vi "Convert Data to Offset values.vi"(11 "Messages":T1(array[cluster])) -> (2 "all values":sgl[](array[numeric]), 3 "Values":string)   [LabVIEW 2025]
uses:
  Station/Controls/Offset_Values.ctl
panel:
  out "Offset F":sgl
  out "Offset E":sgl
  out "Offset D":sgl
  out "Diff Volt F":sgl
  out "Diff Volt E":sgl
  out "Diff Volt D":sgl
  out "Offset A":sgl
  out "Offset B":sgl
  out "Offset C":sgl
  out "Diff Volt C":sgl
  out "Diff Volt B":sgl
  out "Diff Volt A":sgl
  out "OffsetHiBrdgVolt":sgl
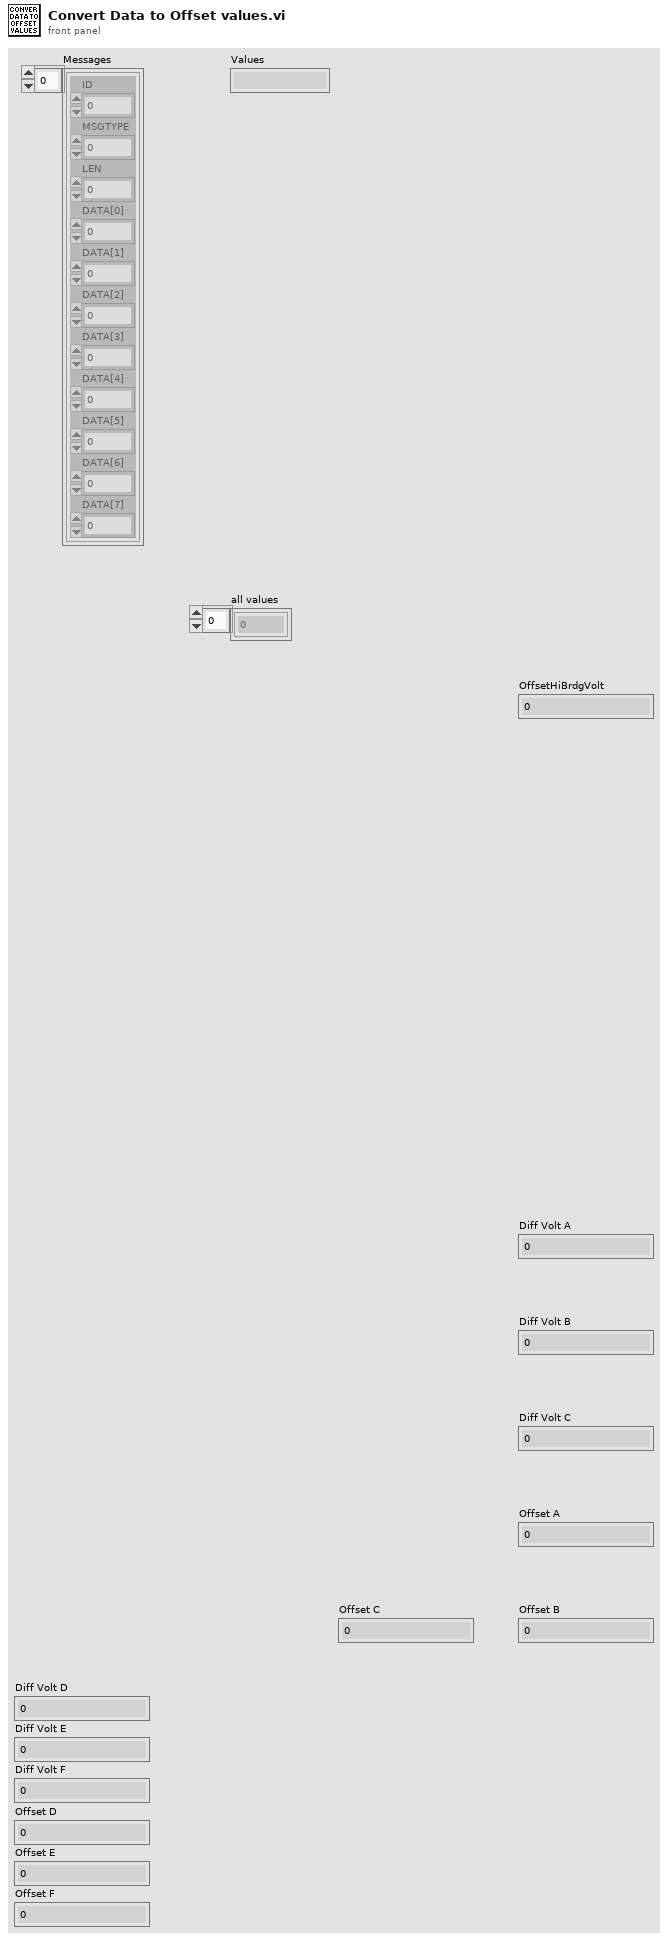
[diagram p1: front panel]
types:
  T1 = cluster{"ID":u32, "MSGTYPE":u8, "LEN":u8, "DATA[0]":u8, "DATA[1]":u8, "DATA[2]":u8, "DATA[3]":u8, "DATA[4]":u8, "DATA[5]":u8, "DATA[6]":u8, "DATA[7]":u8}[]
  T2 = cluster{"ID":u32, "MSGTYPE":u8, "LEN":u8, "DATA[0]":u8, "DATA[1]":u8, "DATA[2]":u8, "DATA[3]":u8, "DATA[4]":u8, "DATA[5]":u8, "DATA[6]":u8, "DATA[7]":u8}
  T3 = typedef "Offset_Values.ctl" = cluster{"OffsetHiBrdgVolt":sgl, "Diff Volt A ":sgl, "Diff Volt B":sgl, "Diff Volt C":sgl, "Diff Volt D":sgl, "Diff Volt E":sgl, "Diff Volt F":sgl, "Offset A":sgl, "Offset B":sgl, "Offset C":sgl, "Offset D":sgl, "Offset E":sgl, "Offset F":sgl}
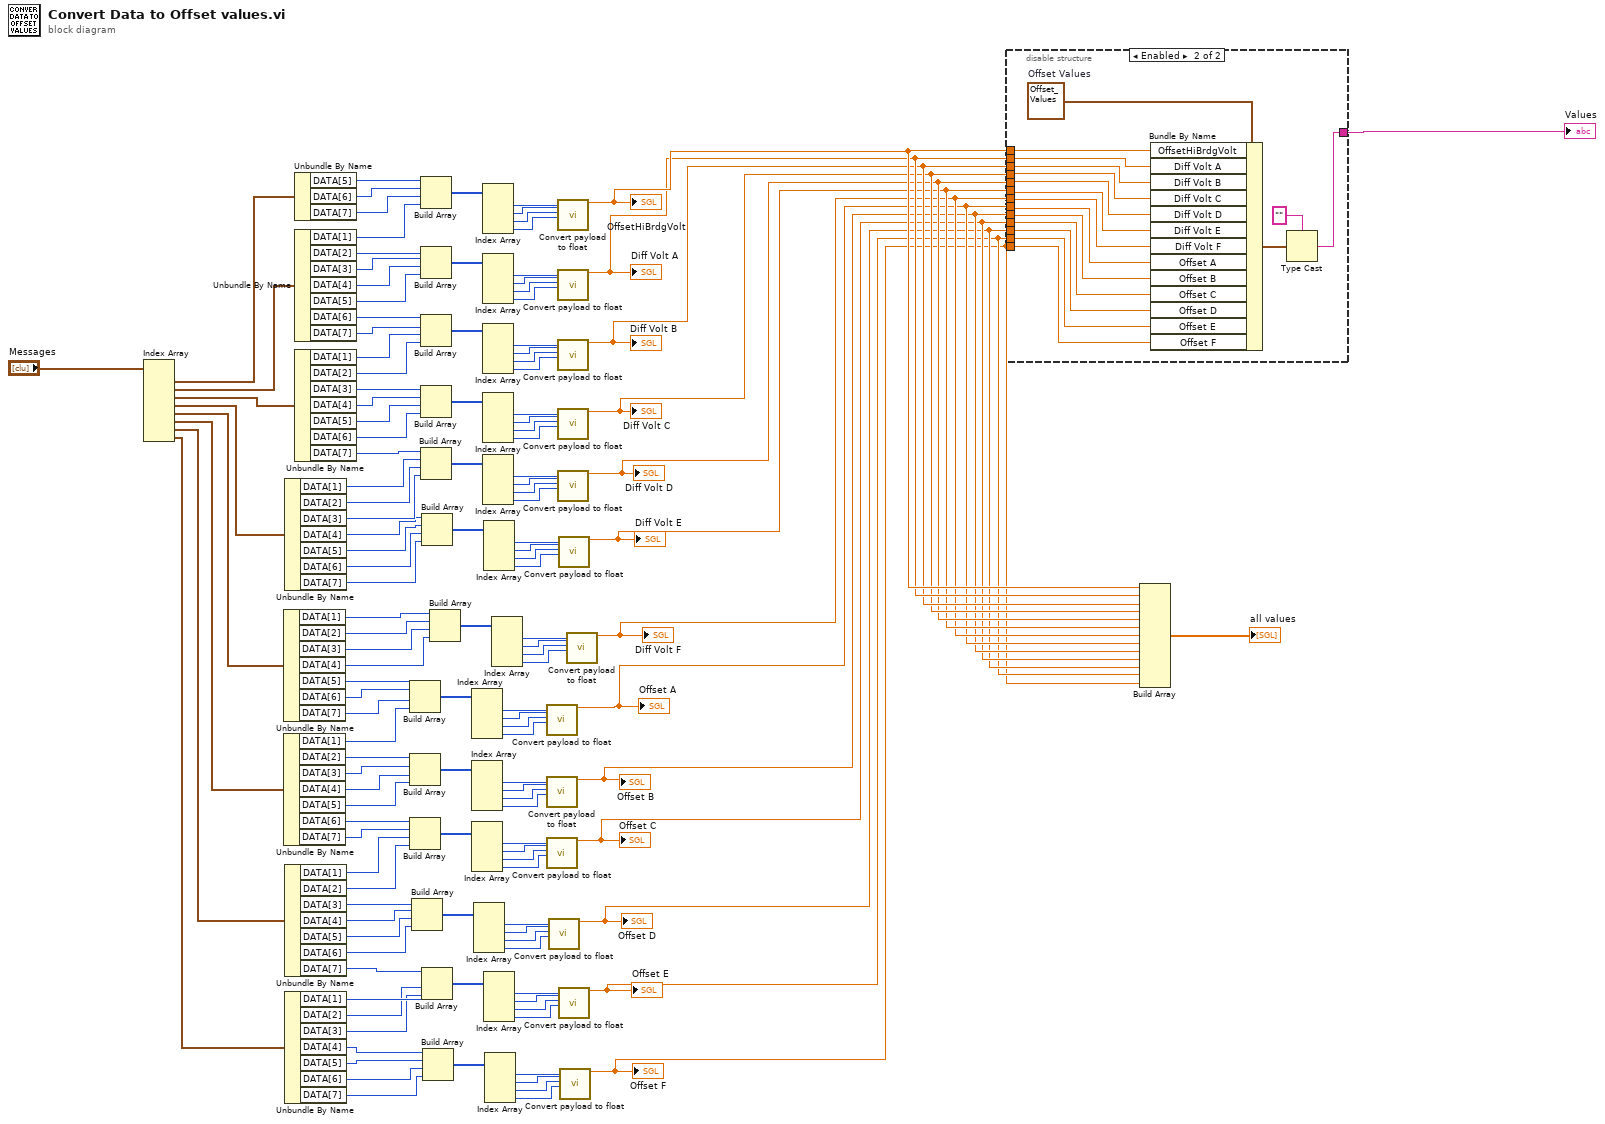
[diagram p0: block diagram]
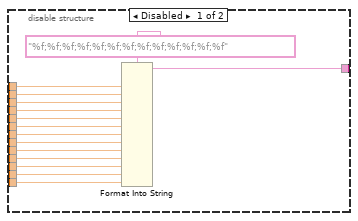
[diagram p2: hidden frame]
diagram:
  n1 = Index Array(array="Messages") -> (element #1=w140:T2, element #2=w139:T2, element #3=w138:T2, element #4=w71:T2, element #5=w137:T2, element #6=w136:T2, element #7=w135:T2, element #8=w34:T2)  [unwired: 8 in]
  n2 = Unbundle By Name(w137) -> ("DATA[1]"=w47:u8, "DATA[2]"=w46:u8, "DATA[3]"=w45:u8, "DATA[4]"=w44:u8, "DATA[5]"=w118:u8, "DATA[6]"=w117:u8, "DATA[7]"=w116:u8)
  n3 = Unbundle By Name(w136) -> ("DATA[1]"=w115:u8, "DATA[2]"=w114:u8, "DATA[3]"=w113:u8, "DATA[4]"=w112:u8, "DATA[5]"=w111:u8, "DATA[6]"=w110:u8, "DATA[7]"=w109:u8)
  n4 = Unbundle By Name(w71) -> ("DATA[1]"=w59:u8, "DATA[2]"=w58:u8, "DATA[3]"=w57:u8, "DATA[4]"=w56:u8, "DATA[5]"=w55:u8, "DATA[6]"=w54:u8, "DATA[7]"=w53:u8)
  n5 = Unbundle By Name(w135) -> ("DATA[1]"=w108:u8, "DATA[2]"=w107:u8, "DATA[3]"=w38:u8, "DATA[4]"=w37:u8, "DATA[5]"=w36:u8, "DATA[6]"=w35:u8, "DATA[7]"=w28:u8)
  n6 = Unbundle By Name(w34) -> ("DATA[1]"=w27:u8, "DATA[2]"=w26:u8, "DATA[3]"=w25:u8, "DATA[4]"=w19:u8, "DATA[5]"=w18:u8, "DATA[6]"=w17:u8, "DATA[7]"=w16:u8)
  n7 = Unbundle By Name(w140) -> ("DATA[5]"=w134:u8, "DATA[6]"=w133:u8, "DATA[7]"=w132:u8)
  n8 = Unbundle By Name(w139) -> ("DATA[1]"=w131:u8, "DATA[2]"=w130:u8, "DATA[3]"=w129:u8, "DATA[4]"=w128:u8, "DATA[5]"=w127:u8, "DATA[6]"=w126:u8, "DATA[7]"=w125:u8)
  n9 = Unbundle By Name(w138) -> ("DATA[1]"=w124:u8, "DATA[2]"=w123:u8, "DATA[3]"=w122:u8, "DATA[4]"=w121:u8, "DATA[5]"=w120:u8, "DATA[6]"=w119:u8, "DATA[7]"=w60:u8)
  n10 = Build Array(w118, w117, w116, w115) -> (w84:u8[])
  n11 = Build Array(w114, w113, w112, w111) -> (w81:u8[])
  n12 = Build Array(w110, w109, w108, w107) -> (w78:u8[])
  n13 = Build Array(w38, w37, w36, w35) -> (w41:u8[])
  n14 = Build Array(w134, w133, w132, w131) -> (w106:u8[])
  n15 = Build Array(w130, w129, w128, w127) -> (w97:u8[])
  n16 = Build Array(w126, w125, w124, w123) -> (w92:u8[])
  n17 = Build Array(w122, w121, w120, w119) -> (w87:u8[])
  n18 = Build Array(w60, w59, w58, w57) -> (w66:u8[])
  n19 = Build Array(w56, w55, w54, w53) -> (w65:u8[])
  n20 = Build Array(w28, w27, w26, w25) -> (w31:u8[])
  n21 = Build Array(w19, w18, w17, w16) -> (w22:u8[])
  n22 = Build Array(w47, w46, w45, w44) -> (w48:u8[])
  n23 = Index Array(array=w84) -> (element #1=w73:u8, element #2=w72:u8, element #3=w86:u8, element #4=w85:u8)  [unwired: 4 in]
  n24 = Index Array(array=w81) -> (element #1=w75:u8, element #2=w74:u8, element #3=w82:u8, element #4=w83:u8)  [unwired: 4 in]
  n25 = Index Array(array=w78) -> (element #1=w77:u8, element #2=w76:u8, element #3=w80:u8, element #4=w79:u8)  [unwired: 4 in]
  n26 = Index Array(array=w41) -> (element #1=w42:u8, element #2=w43:u8, element #3=w39:u8, element #4=w40:u8)  [unwired: 4 in]
  n27 = Index Array(array=w106) -> (element #1=w105:u8, element #2=w104:u8, element #3=w103:u8, element #4=w102:u8)  [unwired: 4 in]
  n28 = Index Array(array=w97) -> (element #1=w98:u8, element #2=w99:u8, element #3=w100:u8, element #4=w101:u8)  [unwired: 4 in]
  n29 = Index Array(array=w92) -> (element #1=w96:u8, element #2=w95:u8, element #3=w94:u8, element #4=w93:u8)  [unwired: 4 in]
  n30 = Index Array(array=w87) -> (element #1=w88:u8, element #2=w89:u8, element #3=w90:u8, element #4=w91:u8)  [unwired: 4 in]
  n31 = Index Array(array=w66) -> (element #1=w70:u8, element #2=w69:u8, element #3=w68:u8, element #4=w67:u8)  [unwired: 4 in]
  n32 = Index Array(array=w65) -> (element #1=w61:u8, element #2=w62:u8, element #3=w63:u8, element #4=w64:u8)  [unwired: 4 in]
  n33 = Index Array(array=w31) -> (element #1=w30:u8, element #2=w29:u8, element #3=w33:u8, element #4=w32:u8)  [unwired: 4 in]
  n34 = Index Array(array=w22) -> (element #1=w23:u8, element #2=w24:u8, element #3=w20:u8, element #4=w21:u8)  [unwired: 4 in]
  n35 = Index Array(array=w48) -> (element #1=w52:u8, element #2=w51:u8, element #3=w50:u8, element #4=w49:u8)  [unwired: 4 in]
  n36 = call "Convert payload to float.vi"("Byte1"=w73, "Byte2"=w72, "Byte3"=w86, "Byte4"=w85) -> ("FloatNumber"=w8:sgl)  [unwired: 15 in]
  "Offset A" <- w8
  n37 = call "Convert payload to float.vi"("Byte1"=w75, "Byte2"=w74, "Byte3"=w82, "Byte4"=w83) -> ("FloatNumber"=w7:sgl)  [unwired: 15 in]
  "Offset B" <- w7
  n38 = call "Convert payload to float.vi"("Byte1"=w77, "Byte2"=w76, "Byte3"=w80, "Byte4"=w79) -> ("FloatNumber"=w6:sgl)  [unwired: 15 in]
  "Offset C" <- w6
  n39 = call "Convert payload to float.vi"("Byte1"=w42, "Byte2"=w43, "Byte3"=w39, "Byte4"=w40) -> ("FloatNumber"=w5:sgl)  [unwired: 15 in]
  "Offset D" <- w5
  n40 = call "Convert payload to float.vi"("Byte1"=w105, "Byte2"=w104, "Byte3"=w103, "Byte4"=w102) -> ("FloatNumber"=w15:sgl)  [unwired: 15 in]
  "OffsetHiBrdgVolt" <- w15
  n41 = call "Convert payload to float.vi"("Byte1"=w98, "Byte2"=w99, "Byte3"=w100, "Byte4"=w101) -> ("FloatNumber"=w14:sgl)  [unwired: 15 in]
  "Diff Volt A" <- w14
  n42 = call "Convert payload to float.vi"("Byte1"=w96, "Byte2"=w95, "Byte3"=w94, "Byte4"=w93) -> ("FloatNumber"=w13:sgl)  [unwired: 15 in]
  "Diff Volt B" <- w13
  n43 = call "Convert payload to float.vi"("Byte1"=w88, "Byte2"=w89, "Byte3"=w90, "Byte4"=w91) -> ("FloatNumber"=w12:sgl)  [unwired: 15 in]
  "Diff Volt C" <- w12
  n44 = call "Convert payload to float.vi"("Byte1"=w70, "Byte2"=w69, "Byte3"=w68, "Byte4"=w67) -> ("FloatNumber"=w11:sgl)  [unwired: 15 in]
  "Diff Volt D" <- w11
  n45 = call "Convert payload to float.vi"("Byte1"=w61, "Byte2"=w62, "Byte3"=w63, "Byte4"=w64) -> ("FloatNumber"=w10:sgl)  [unwired: 15 in]
  "Diff Volt E" <- w10
  n46 = call "Convert payload to float.vi"("Byte1"=w30, "Byte2"=w29, "Byte3"=w33, "Byte4"=w32) -> ("FloatNumber"=w4:sgl)  [unwired: 15 in]
  "Offset E" <- w4
  n47 = call "Convert payload to float.vi"("Byte1"=w23, "Byte2"=w24, "Byte3"=w20, "Byte4"=w21) -> ("FloatNumber"=w3:sgl)  [unwired: 15 in]
  "Offset F" <- w3
  n48 = call "Convert payload to float.vi"("Byte1"=w52, "Byte2"=w51, "Byte3"=w50, "Byte4"=w49) -> ("FloatNumber"=w9:sgl)  [unwired: 15 in]
  "Diff Volt F" <- w9
  n49 = disable-structure shown="Enabled" {
    disable-tunnel: w15 -> [w155 w172]
    disable-tunnel: w14 -> [w154 w171]
    disable-tunnel: w13 -> [w153 w170]
    disable-tunnel: w12 -> [w152 w169]
    disable-tunnel: w11 -> [w151 w168]
    disable-tunnel: w10 -> [w150 w167]
    disable-tunnel: w9 -> [w149 w166]
    disable-tunnel: w8 -> [w148 w165]
    disable-tunnel: w7 -> [w147 w164]
    disable-tunnel: w6 -> [w146 w163]
    disable-tunnel: w5 -> [w145 w162]
    disable-tunnel: w4 -> [w144 w161]
    disable-tunnel: w3 -> [w143 w160]
    disable-tunnel: [w142 w158] -> w2
    frame Disabled {
      n50 = Format Into String(format string="%f;%f;%f;%f;%f;%f;%f;%f;%f;%f;%f;%f;%f", w155, w154, w153, w152, w151, w150, w149, w148, w147, w146, w145, w144, w143) -> (resulting string=w142:string)  [unwired: 2 in, 1 out]
    }
    frame Enabled {
      w173 = T3 {"OffsetHiBrdgVolt"=0.0, "Diff Volt A "=0.0, "Diff Volt B"=0.0, "Diff Volt C"=0.0, "Diff Volt D"=0.0, "Diff Volt E"=0.0, "Diff Volt F"=0.0, "Offset A"=0.0, "Offset B"=0.0, "Offset C"=0.0, "Offset D"=0.0, "Offset E"=0.0, "Offset F"=0.0}  # Offset Values
      n51 = Bundle By Name(cluster=w173, "OffsetHiBrdgVolt"=w172, "Diff Volt A"=w171, "Diff Volt B"=w170, "Diff Volt C"=w169, "Diff Volt D"=w168, "Diff Volt E"=w167, "Diff Volt F"=w166, "Offset A"=w165, "Offset B"=w164, "Offset C"=w163, "Offset D"=w162, "Offset E"=w161, "Offset F"=w160) -> (w159:T3)
      n52 = Type Cast(type="", x=w159) -> (*(type *) &x=w158:string)
    }
  }
  "Values" <- w2
  n53 = Build Array(w15, w14, w13, w12, w11, w10, w9, w8, w7, w6, w5, w4, w3) -> (→"all values":sgl[])
